vi "编码判断.vi"(8 "错误输入":errorcluster, 10 "编码规则":string[](array[string]), 11 "输入编码":string) -> (0 "错误输出":errorcluster, 2 "输出编码":string, 3 "有效编码？":bool)   [LabVIEW 2020]
uses:
  <vilib>/regexp/Match Regular Expression.xnode
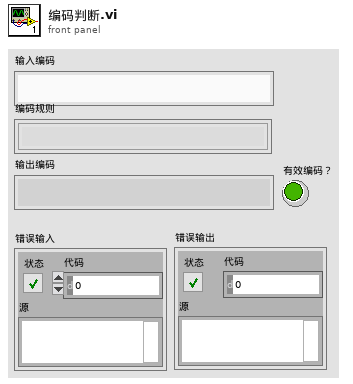
[diagram p1: front panel]
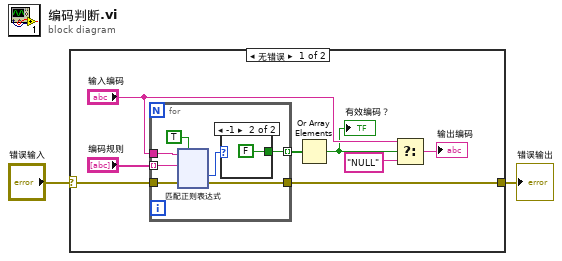
[diagram p0: block diagram]
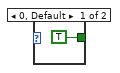
[diagram p2: hidden frame]
diagram:
  n1 = case shown="无错误" "错误输入" {
    selector: "错误输入" -> [w4 w131]
    tunnel: [w3 w131] -> w1
    frame No Error {
      n2 = for {
        tunnel: "输入编码" -> [w17]
        tunnel: "编码规则" -> [w15] mode=indexing
        tunnel: [w14] -> w9 mode=indexing
        tunnel: w4 -> [w13]
        tunnel: [w12] -> w3
        n3 = xnode "匹配正则表达式"("输入字符串"=w17, "正则表达式"=w15, "错误输入"=w13, "忽略大小写？(F)"=TRUE) -> ("匹配后偏移量"=w16:i32, "错误输出"=w12:errorcluster)  [unwired: 2 in, 3 out]
        n4 = case shown="-1" w16 {
          tunnel: [TRUE FALSE] -> w14
          frame 0, Default {
          }
          frame -1 {
          }
        }
      }
      n5 = Or Array Elements(Boolean array=w9) -> (logical OR=w6:bool)
      "有效编码？" <- w6
      n6 = Select(t="输入编码", s=w6, f="NULL") -> (s? t:f=→"输出编码":string)
    }
    frame Error {
    }
  }
  "错误输出" <- w1
